vi "Get All Methods.vi"(8 "error in (no error)":errorcluster) -> (0 "error out":errorcluster, 3 "Methods[]":T1(array[cluster]))   [LabVIEW 2023]
panel:
  out "exe time (ms)":u32
  # "After some initial cleanup run time:\n\n70s\n\nAfter a little optimization:\n\n11s"
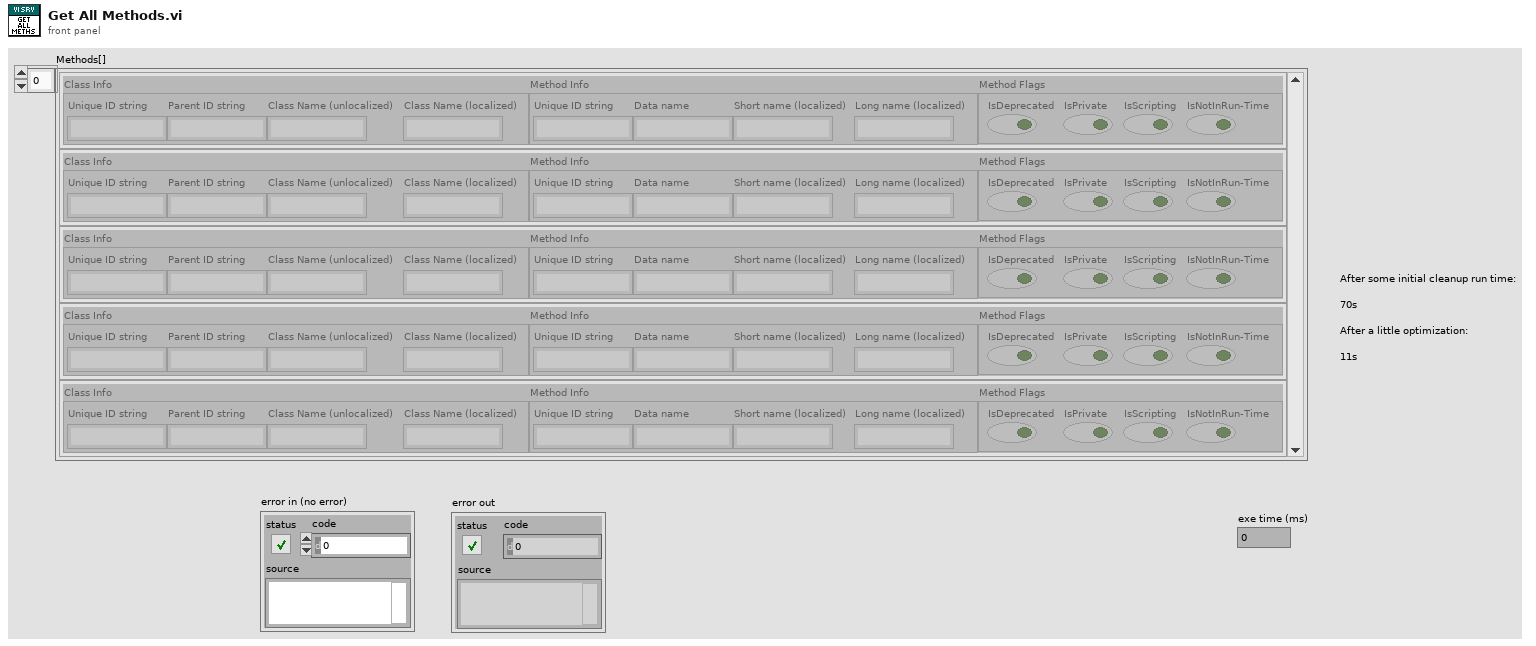
[diagram p1: front panel]
types:
  T1 = cluster{"Class Info":cluster{"Unique ID string":string, "Parent ID string":string, "Class Name (unlocalized)":string, "Class Name (localized)":string}, "Method Info":cluster{"Unique ID string":string, "Data name":string, "Short name (localized)":string, "Long name (localized)":string}, "Method Flags":cluster{"IsDeprecated":bool, "IsPrivate":bool, "IsScripting":bool, "IsNotInRun-Time":bool}}[]
  T2 = cluster{"Unique ID string":string, "Parent ID string":string, "Class Name (unlocalized)":string, "Class Name (localized)":string}[]
  T3 = cluster{"Property/Method Info":cluster{"Unique ID string":string, "Parent ID string":string, "Class Name (unlocalized)":string, "Class Name (localized)":string}, "Property Info":cluster{"Unique ID string":string, "Data name":string, "Short name (localized)":string, "Long name (localized)":string}, "Method Flags":cluster{"IsDeprecated":bool, "IsPrivate":bool, "IsScripting":bool, "IsNotInRun-Time":bool}}[]
  T4 = cluster{"Unique ID string":string, "Data name":string, "Short name (localized)":string, "Long name (localized)":string}[]
  T5 = cluster{"IsDeprecated":bool, "IsPrivate":bool, "IsScripting":bool, "IsNotInRun-Time":bool}
  T6 = cluster{"Property/Method Info":cluster{"Unique ID string":string, "Parent ID string":string, "Class Name (unlocalized)":string, "Class Name (localized)":string}, "Property Info":cluster{"Unique ID string":string, "Data name":string, "Short name (localized)":string, "Long name (localized)":string}, "Method Flags":cluster{"IsDeprecated":bool, "IsPrivate":bool, "IsScripting":bool, "IsNotInRun-Time":bool}}
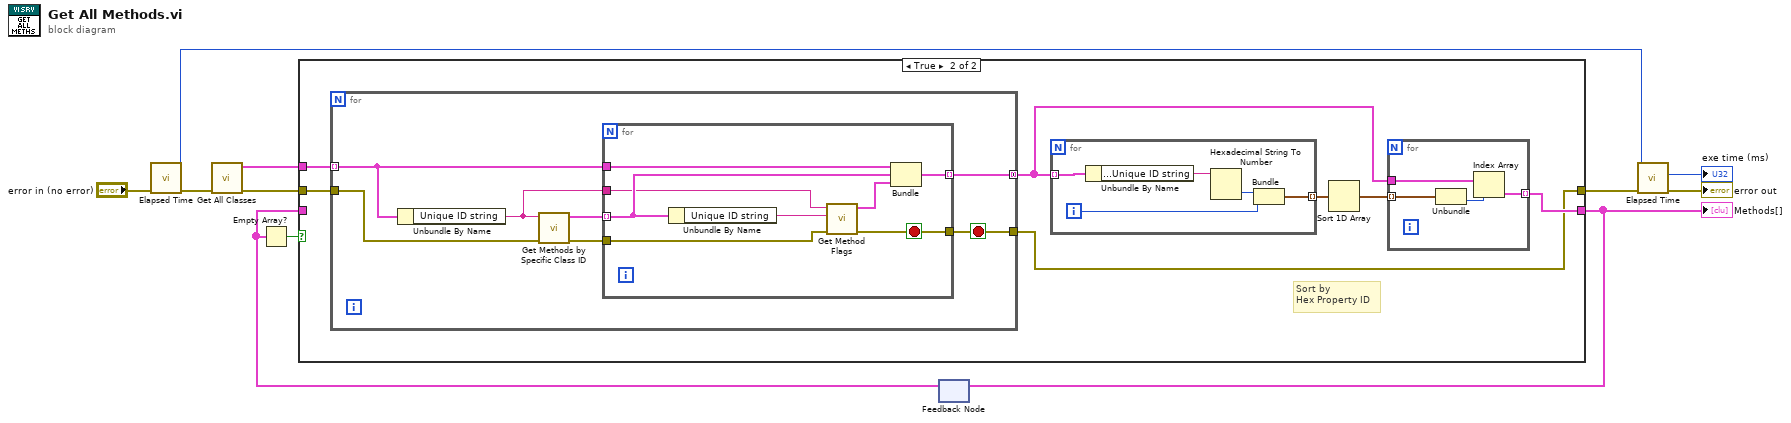
[diagram p0: block diagram]
diagram:
  n1 = call "Elapsed Time.vi"("error in"="error in (no error)") -> ("error out"=w8:errorcluster, "millisecond timer value"=w3:u32)  [unwired: 6 in, 3 out]
  n2 = call "Get All Classes.vi"("error in (no error)"=w8) -> ("error out"=w1:errorcluster, "VI Server Classes[]"=w11:T2)  [unwired: 9 in]
  n3 = feedback #1() -> (w5:T3)  [unwired: 1 in]
  n4 = Empty Array?(array=w5) -> (empty?=w4:bool)
  n5 = case shown="True" w4 {
    tunnel: w11 -> [_ w20]
    tunnel: [w13 w16] -> w10
    tunnel: w5 -> [w13 _]
    tunnel: w1 -> [w12 w15]
    tunnel: [w12 w14] -> w7
    frame False {
    }
    frame True {
      # "Sort by\nHex Property ID"
      n6 = for {
        tunnel: w20 -> [w27] mode=indexing
        tunnel: [w26] -> w17 mode=concatenating
        tunnel: w15 -> [w23]
        tunnel: [w25] -> w14
        stop <- w25 stop-if-true
        n7 = Unbundle By Name(w27) -> ("Unique ID string"=w24:string)
        n8 = call "Get Methods by Specific Class ID.vi"("error in (no error)"=w23, "Class ID"=w24) -> ("error out"=w22:errorcluster, "Methods[]"=w21:T4)  [unwired: 8 in]
        n9 = for {
          tunnel: w21 -> [w34] mode=indexing
          tunnel: w24 -> [w32]
          tunnel: w27 -> [w35]
          tunnel: [w33] -> w26 mode=indexing
          tunnel: w22 -> [w30]
          tunnel: [w28] -> w25
          stop <- w28 stop-if-true
          n10 = Unbundle By Name(w34) -> ("Unique ID string"=w31:string)
          n11 = call "Get Method Flags.vi"("error in (no error)"=w30, "Method ID"=w31, "Class ID"=w32) -> ("error out"=w28:errorcluster, "Method Flags"=w29:T5)  [unwired: 7 in]
          n12 = Bundle("Property/Method Info"=w35, "Property Info"=w34, "Method Flags"=w29) -> (w33:T6)  [unwired: 1 in]
        }
      }
      n13 = for {
        tunnel: [w38] -> w19 mode=indexing
        tunnel: w17 -> [w37] mode=indexing
        i -> [w39]
        n14 = Unbundle By Name(w37) -> ("Property/Method Info.Unique ID string"=w36:string)
        n15 = Hexadecimal String To Number(string=w36) -> (number=w40:u32)  [unwired: 2 in, 1 out]
        n16 = Bundle(w40, w39) -> (w38:cluster{u32, i32})  [unwired: 1 in]
      }
      n17 = Sort 1D Array(array=w19) -> (sorted array=w18:cluster{u32, i32}[])
      n18 = for {
        tunnel: w18 -> [w44] mode=indexing
        tunnel: [w42] -> w16 mode=indexing
        tunnel: w17 -> [w41]
        n19 = Unbundle(w44) -> (w43:i32)  [unwired: 1 out]
        n20 = Index Array(array=w41, index=w43) -> (element=w42:T6)
      }
    }
  }
  "Methods[]" <- w10
  n21 = feedback-in #1(w10) -> ()
  n22 = call "Elapsed Time.vi"("error in"=w7, "past time"=w3) -> ("error out"=→"error out":errorcluster, "elapsed time (ms)"=→"exe time (ms)":u32)  [unwired: 5 in, 3 out]
